vi "escribeRutaClasePruebas.vi"(8 "error in (no error)":errorcluster, 11 "Fabrica de Equipos in":refnum<class "Fabrica de Equipos.lvclass">) -> (0 "error out":errorcluster, 3 "Fabrica de Equipos out":refnum<class "Fabrica de Equipos.lvclass">)   [LabVIEW 2019, in "Fabrica de Equipos.lvclass"]
uses:
  Fabrica de Equipos.lvclass
  Pruebas/Prueba/Prueba.lvclass
panel:
  in  "NombrePruebas":string[](array[string])
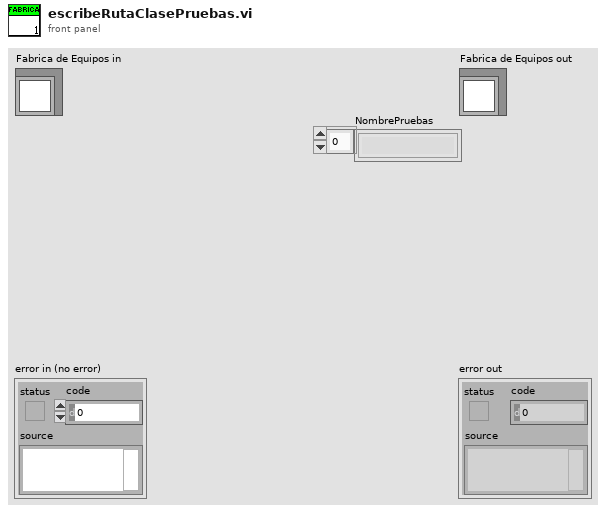
[diagram p1: front panel]
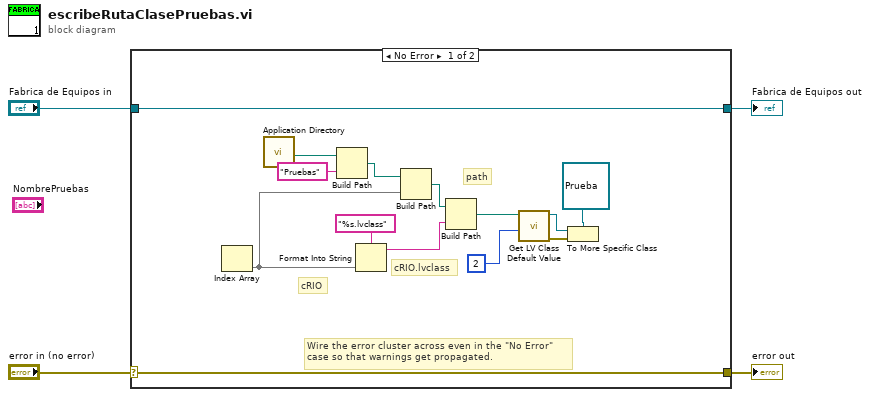
[diagram p0: block diagram]
diagram:
  n1 = case shown="No Error" "error in (no error)" {
    selector: "error in (no error)" -> [w17 w20]
    tunnel: [w17 w20] -> w3
    tunnel: [w18 w19] -> w1
    tunnel: "Fabrica de Equipos in" -> [w18 w19]
    frame No Error {
      # "cRIO.lvclass"
      # "path"
      # "cRIO"
      # "Wire the error cluster across even in the \"No Error\"\ncase so that warnings get propagated."
      n2 = Index Array() -> (element=w11)  [unwired: 2 in]
      n3 = call <vilib>:"Application Directory.vi"() -> ("Application Directory"=w16:path)
      n4 = Build Path(base path=w16, name or relative path="Pruebas") -> (appended path=w14:path)
      n5 = Format Into String(format string="%s.lvclass", w11) -> (resulting string=w10:string)  [unwired: 2 in, 1 out]
      n6 = Build Path(base path=w14, name or relative path=w11) -> (appended path=w13:path)
      n7 = Build Path(base path=w13, name or relative path=w10) -> (appended path=w8:path)
      n8 = call <vilib>:"Get LV Class Default Value.vi"("options"=u32 2, "class path"=w8) -> ("error out"=w7:errorcluster, "object"=w6:refnum<class>)  [unwired: 8 in]
      n9 = To More Specific Class(target class=refnum<class "Prueba.lvclass"> refnum ("Prueba.lvclass"), reference=w6, error in=w7) -> ()  [unwired: 2 out]
    }
    frame Error {
    }
  }
  "error out" <- w3
  "Fabrica de Equipos out" <- w1
